vi "TheShooter.vi"() -> ()   [LabVIEW 2019]
uses:
  <vilib>/Rock Robotics/WPI/ThirdParty/Phoenix-LabVIEW/Motor Controller/Controls/CTRE_Phoenix_MotorControl_ControlMode.ctl
  <vilib>/Rock Robotics/WPI/Utilities/WPI_GetSetVariantRefNum.vi
  Robot Global Data.vi
  <vilib>/Rock Robotics/Network Tables/NT Read Number.vi
  <vilib>/Rock Robotics/WPI/ThirdParty/Phoenix-LabVIEW/Motor Controller/Get/CTRE_Phoenix_MotorController_IntegratedSensorData_TalonFX.vi
panel:
  out "shoot state":dbl
  out "Waveform Chart":dbl(graph)
  out "Position":dbl format="%.2f"
  out "MVelocity":dbl
  out "WVelocity":dbl
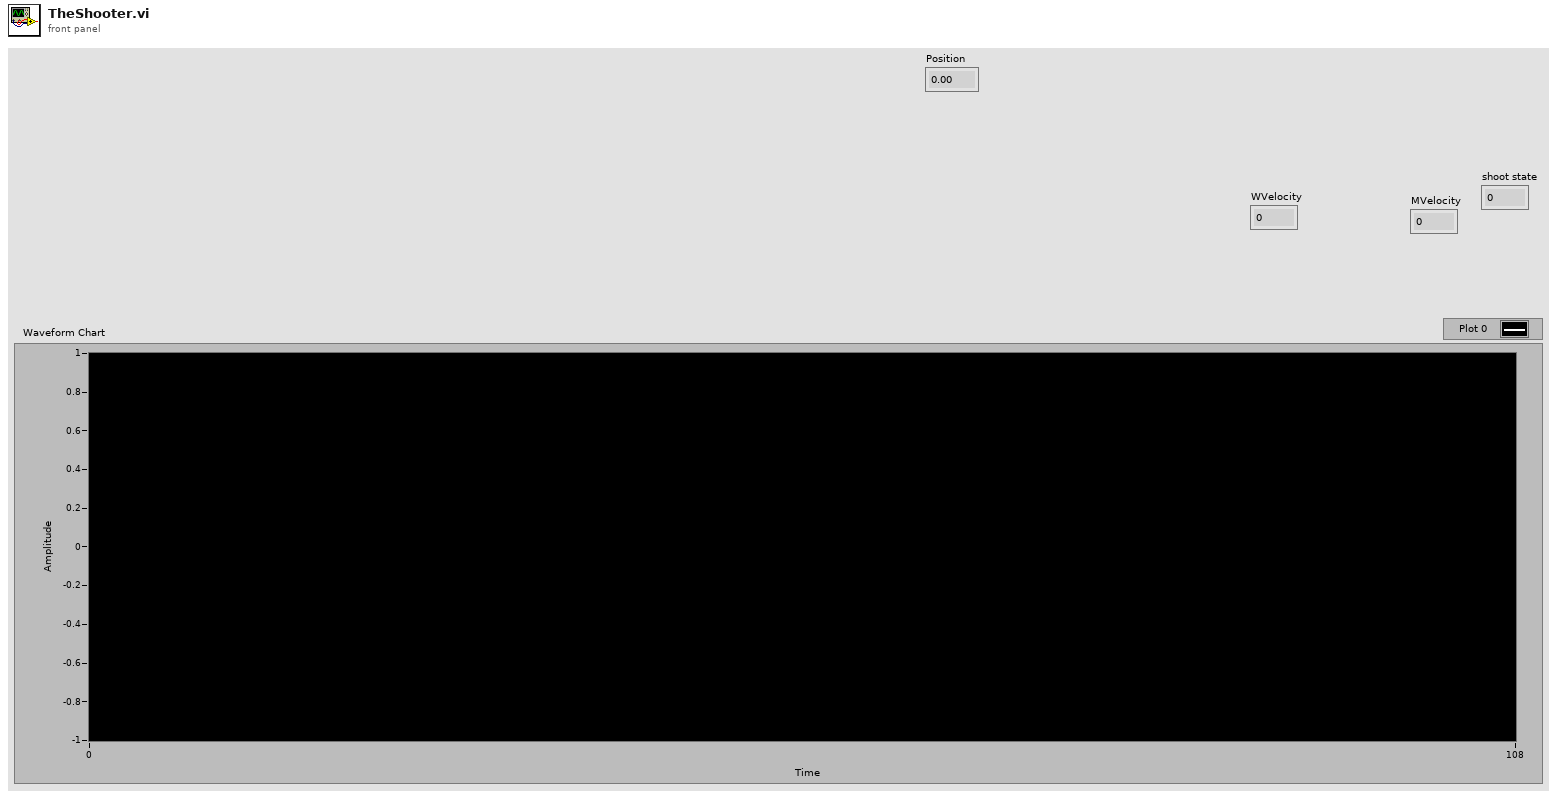
[diagram p1: front panel]
types:
  T1 = typedef "WPI_MotorControlDeviceRef.ctl" = cluster{"DeviceStatus":errorcluster, "Type":T2, "PWM":cluster{"PWM Channel":T3, "DeadBand":T4}, "CAN":cluster{"Device Number":u8, "SetOutput VI Ref":variant, "GetOutput VI Ref":variant, "Enable VI Ref":variant, "Disable VI Ref":variant, "Data":variant}, "Invert":bool, "DIO PWM":cluster{"PWM \"Enable\" Channel":T3, "DIOChannel":T5, "PWM Rate":dbl}}
  T2 = typedef "WPI_MotorControlType.ctl" = enum16{"PWM", "CAN", "DIO PWM"}
  T3 = typedef "FPGA_DIOPWMChannel.ctl" = enum8{"PWM 0", "PWM 1", "PWM 2", "PWM 3", "PWM 4", "PWM 5", "PWM 6", "PWM 7", "PWM 8", "PWM 9", "PWM MXP 0", "PWM MXP 1", "PWM MXP 2", "PWM MXP 3", "PWM MXP 4", "PWM MXP 5", "PWM MXP 6", "PWM MXP 7", "PWM MXP 8", "PWM MXP 9", "Invalid"}
  T4 = typedef "WPI_PWMDeadband.ctl" = cluster{"Name":string, "maxPositivePwm":i32, "minPositivePwm":i32, "centerPwm":i32, "maxNegativePwm":i32, "minNegativePwm":i32, "angularRange":u16}
  T5 = typedef "FPGA_DIOChannel.ctl" = enum8{"DIO 0", "DIO 1", "DIO 2", "DIO 3", "DIO 4", "DIO 5", "DIO 6", "DIO 7", "DIO 8", "DIO 9", "DIO MXP 0", "DIO MXP 1", "DIO MXP 2", "DIO MXP 3", "DIO MXP 4", "DIO MXP 5", "DIO MXP 6", "DIO MXP 7", "DIO MXP 8", "DIO MXP 9", "DIO MXP 10", "DIO MXP 11", "DIO MXP 12", "DIO MXP 13", "DIO MXP 14", "DIO MXP 15", "SPI Port CS1", "SPI Port CS2", "SPI Port CS3", "SPI Port MISO", "SPI Port MOSI", "Invalid"}
  T6 = typedef "WPI_JoystickDevRef.ctl" = cluster{"Device":T7}
  T7 = typedef "WPI_JoystickDeviceEnum.ctl" = enum16{"USB 0", "USB 1", "USB 2", "USB 3", "USB 4", "USB 5"}
  T8 = typedef "CTRE_Phoenix_MotorControl_ControlMode.ctl" = u16
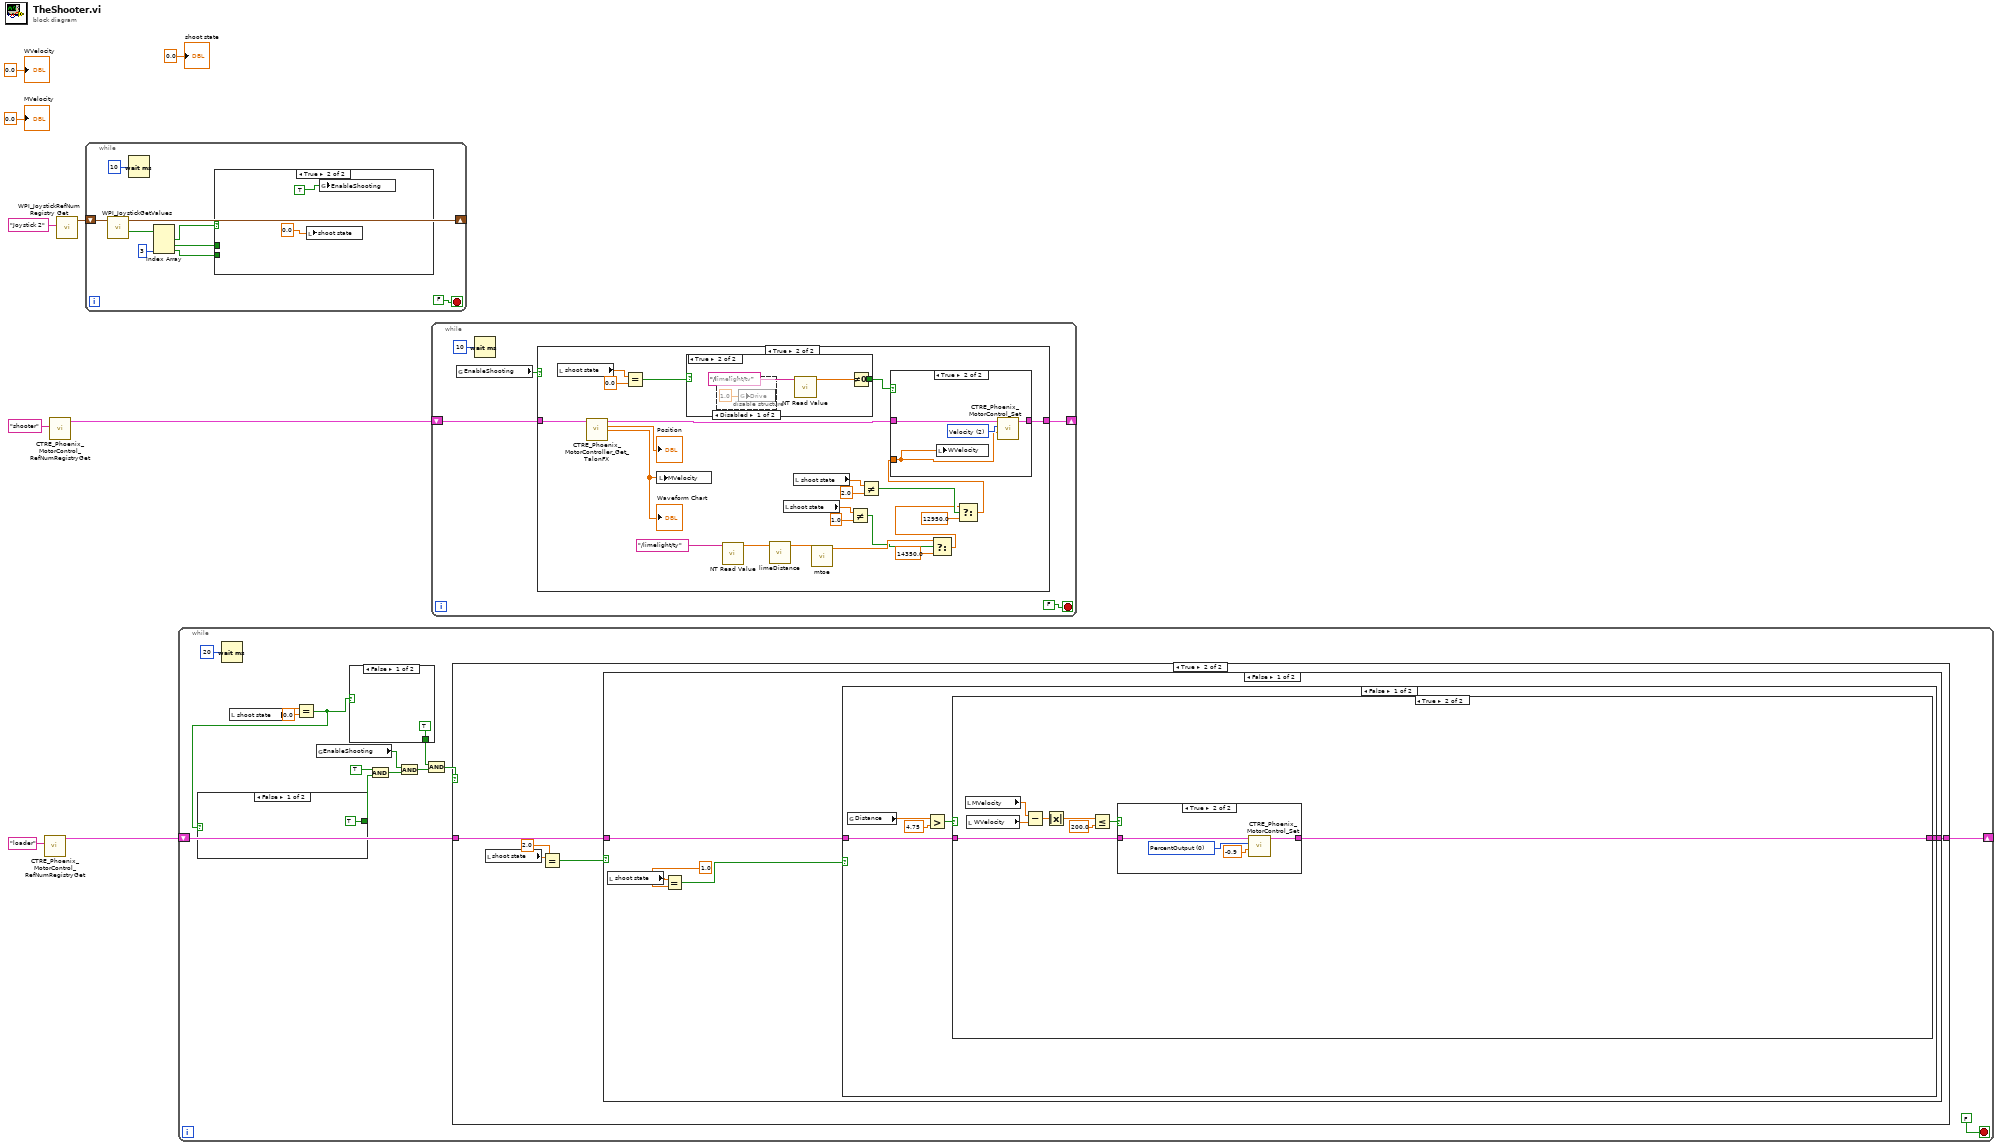
[diagram p0: block diagram]
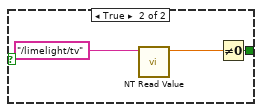
[diagram p2: hidden frame]
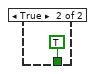
[diagram p3: hidden frame]
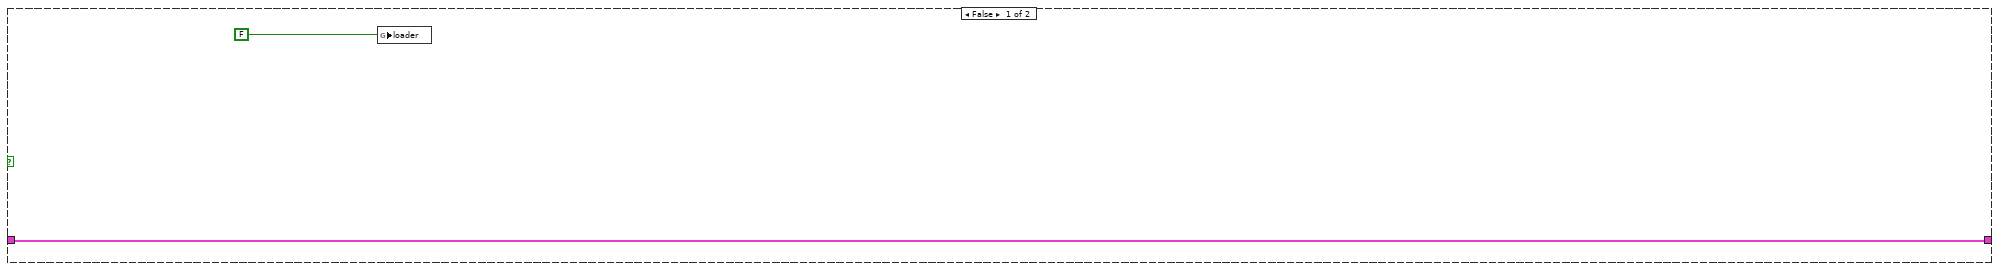
[diagram p4: hidden frame]
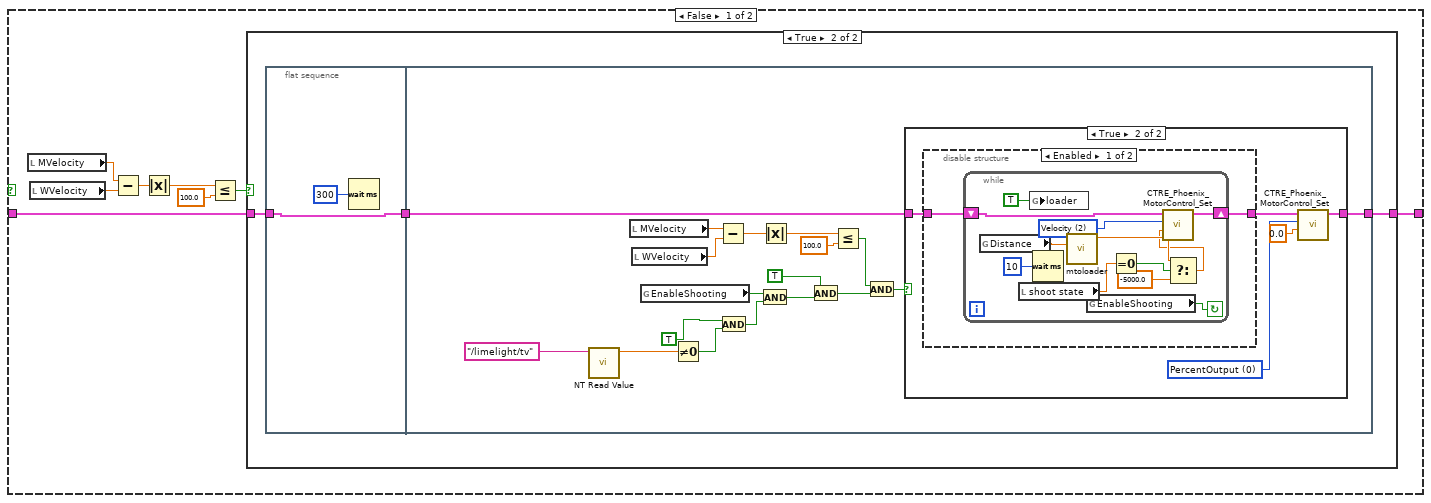
[diagram p5: hidden frame]
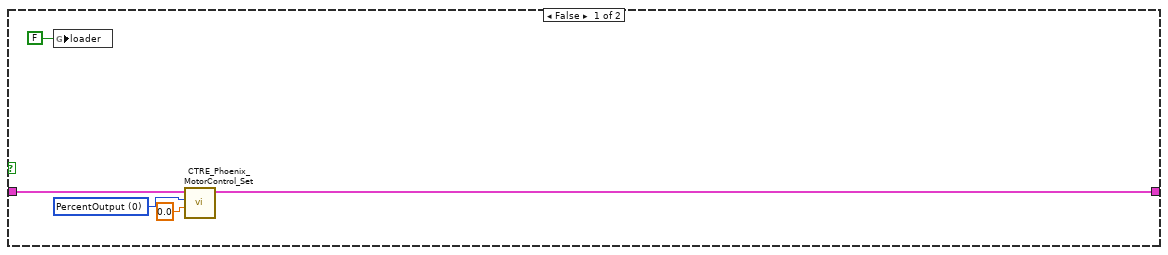
[diagram p6: hidden frame]
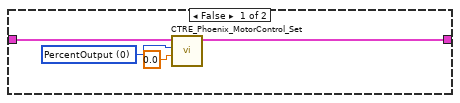
[diagram p7: hidden frame]
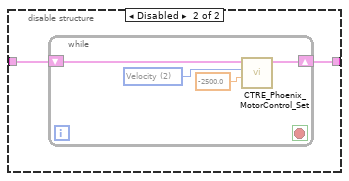
[diagram p8: hidden frame]
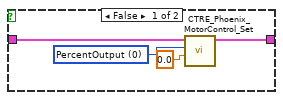
[diagram p9: hidden frame]
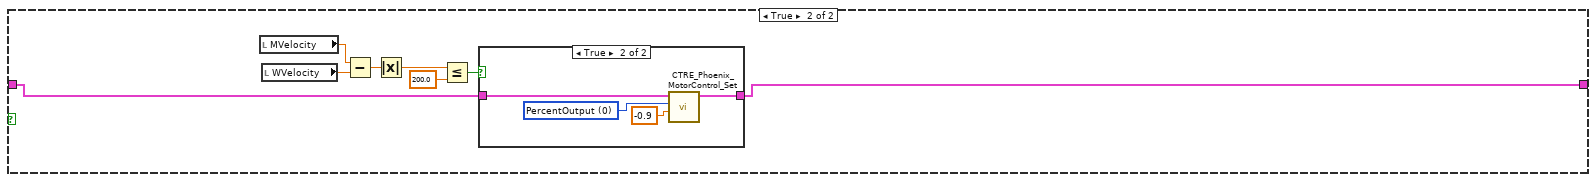
[diagram p10: hidden frame]
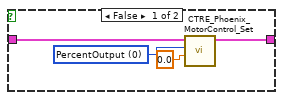
[diagram p11: hidden frame]
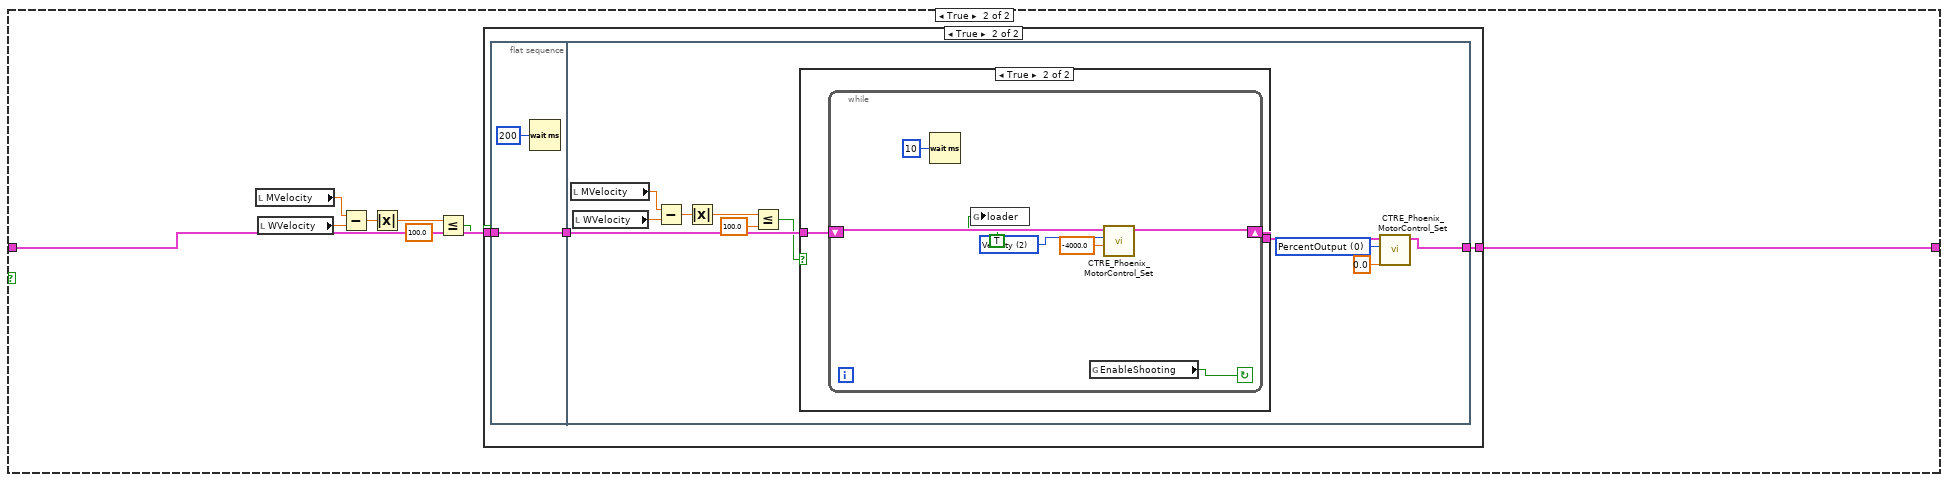
[diagram p12: hidden frame]
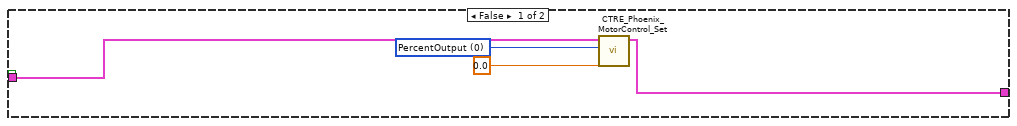
[diagram p13: hidden frame]
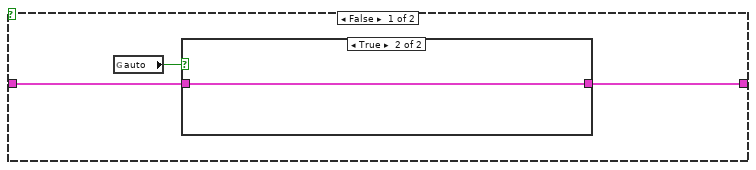
[diagram p15: hidden frame]
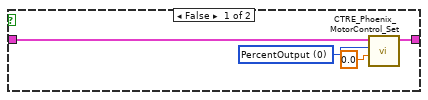
[diagram p16: hidden frame]
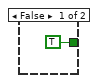
[diagram p17: hidden frame]
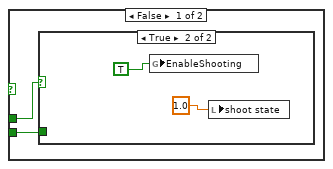
[diagram p20: hidden frame]
diagram:
  n1 = call <vilib>:"CTRE_Phoenix_MotorControl_RefNumRegistryGet.vi"("refnum name"="loader") -> ("PhoenixMotorControlDevRef"=w3:T1)  [unwired: 9 in, 1 out]
  n2 = call <vilib>:"CTRE_Phoenix_MotorControl_RefNumRegistryGet.vi"("refnum name"="shooter") -> ("PhoenixMotorControlDevRef"=w7:T1)  [unwired: 9 in, 1 out]
  n3 = call <vilib>:"WPI_JoystickRefNum Registry Get.vi"("refnum name"="Joystick 2") -> ("JoystickDevRef"=w2:T6)  [unwired: 9 in, 1 out]
  n4 = while {
    shift-right: [w13] -> _
    shift-left: w2 -> [w15]
    stop <- FALSE stop-if-true
    n5 = call <vilib>:"WPI_JoystickGetValues.vi"("JoystickDevRef"=w15) -> ("Buttons"=w18:bool[], "JoystickDevRef"=w13:T6)  [unwired: 6 in, 3 out]
    n6 = Wait (ms)(milliseconds to wait=u32 10) -> ()  [unwired: 1 out]
    n7 = Index Array(array=w18, index #3=3 ("index")) -> (element #1=w12:bool, element #2=w11:bool, element #3=w10:bool)  [unwired: 2 in]
    n8 = case shown="True" w12 {
      tunnel: w11 -> [w20 _]
      tunnel: w10 -> [w19 _]
      frame False {
        n9 = case shown="True" w20 {
          tunnel: w19 -> [w21 _]
          frame False {
            n10 = case shown="True" w21 {
              frame False {
                n11 = global read "Robot Global Data.vi" "auto"() -> (w22:bool)
                n12 = case shown="False" w22 {
                  frame False {
                    n13 = global write "Robot Global Data.vi" "EnableShooting"(FALSE ("EnableShooting")) -> ()
                  }
                  frame True {
                  }
                }
              }
              frame True {
                n14 = global write "Robot Global Data.vi" "EnableShooting"(TRUE ("EnableShooting")) -> ()
                n15 = local write "shoot state"(2.0 ("Loader")) -> ()
              }
            }
          }
          frame True {
            n16 = global write "Robot Global Data.vi" "EnableShooting"(TRUE ("EnableShooting")) -> ()
            n17 = local write "shoot state"(1.0 ("Loader")) -> ()
          }
        }
      }
      frame True {
        n18 = local write "shoot state"(0.0 ("Loader")) -> ()
        n19 = global write "Robot Global Data.vi" "EnableShooting"(TRUE ("EnableShooting")) -> ()
      }
    }
  }
  n20 = while {
    shift-right: [w41] -> _
    shift-left: w3 -> [w42]
    stop <- FALSE stop-if-true
    n21 = Wait (ms)(milliseconds to wait=u32 20) -> ()  [unwired: 1 out]
    n22 = local read "shoot state"() -> (w33:dbl)
    n23 = Equal?(x=w33, y=0.0) -> (x = y?=w31:bool)
    n24 = case shown="False" w31 {
      tunnel: [TRUE w45] -> w35
      frame False {
      }
      frame True {
        n25 = call-poly <vilib>:"NT Read Value.vi"("Name"="/limelight/tv") -> ("Numeric"=w46:dbl)  [unwired: 9 in, 1 out]
        n26 = Not Equal To 0?(x=w46) -> (x != 0?=w45:bool)
      }
    }
    n27 = global read "Robot Global Data.vi" "EnableShooting"() -> (w37:bool)
    n28 = case shown="False" w31 {
      tunnel: [TRUE ("In Angle") TRUE ("In Angle")] -> w38
      frame False {
      }
      frame True {
      }
    }
    n29 = And(x=TRUE, y=w35) -> (x .and. y?=w34:bool)
    n30 = And(x=w37, y=w34) -> (x .and. y?=w36:bool)
    n31 = And(x=w38, y=w36) -> (x .and. y?=w39:bool)
    n32 = case shown="True" w39 {
      tunnel: w42 -> [w51 w55]
      tunnel: [w51 w56] -> w41
      frame False {
        n33 = global write "Robot Global Data.vi" "loader"(FALSE ("If loaderMoves")) -> ()
      }
      frame True {
        n34 = local read "shoot state"() -> (w54:dbl)
        n35 = Equal?(x=w54, y=2.0) -> (x = y?=w52:bool)
        n36 = case shown="False" w52 {
          tunnel: [w61 w170] -> w56
          tunnel: w55 -> [w60 w171]
          frame False {
            n37 = local read "shoot state"() -> (w59:dbl)
            n38 = Equal?(x=w59, y=1.0) -> (x = y?=w57:bool)
            n39 = case shown="False" w57 {
              tunnel: [w66 w148] -> w61
              tunnel: w60 -> [w65 w149]
              frame False {
                n40 = global read "Robot Global Data.vi" "Distance"() -> (w64:dbl)
                n41 = Greater?(x=w64, y=4.75) -> (0:w62:bool)
                n42 = case shown="True" w62 {
                  tunnel: [w69 w132] -> w66
                  tunnel: w65 -> [w67 w133]
                  frame False {
                    n43 = local read "MVelocity"() -> (w73:dbl)
                    n44 = local read "WVelocity"() -> (w72:dbl)
                    n45 = Subtract(x=w73, y=w72) -> (x-y=w71:dbl)
                    n46 = Absolute Value(x=w71) -> (abs(x)=w70:dbl)
                    n47 = Less Or Equal?(x=w70, y=100.0) -> (x <= y?=w68:bool)
                    n48 = case shown="True" w68 {
                      tunnel: w67 -> [w77 w82]
                      tunnel: [w76 w81] -> w69
                      frame False {
                        w79 = T8 0 items=["PercentOutput"=0, "Position"=1, "Velocity"=2, "Current"=3, "Follower"=5, "MotionProfile"=6, "MotionMagic"=7, "MotionProfileArc"=10, "Disabled"=15] ("Control Mode")
                        n49 = global write "Robot Global Data.vi" "loader"(FALSE ("If loaderMoves")) -> ()
                        n50 = call <vilib>:"CTRE_Phoenix_MotorControl_Set.vi"("Output"=0.0, "Control Mode"=w79, "PhoenixMotorControlDevRef"=w77) -> ("PhoenixMotorControlDevRef"=w76:T1)  [unwired: 7 in, 1 out]
                      }
                      frame True {
                        n51 = flat-sequence {
                          tunnel: w82 -> [w84]
                          tunnel: [w84] -> w80
                          tunnel: [w101] -> w81
                          tunnel: w80 -> [w102]
                          frame #0 {
                            n52 = Wait (ms)(milliseconds to wait=u32 300) -> ()  [unwired: 1 out]
                          }
                          frame #1 {
                            n53 = call-poly <vilib>:"NT Read Value.vi"("Name"="/limelight/tv") -> ("Numeric"=w90:dbl)  [unwired: 9 in, 1 out]
                            n54 = local read "MVelocity"() -> (w97:dbl)
                            n55 = local read "WVelocity"() -> (w98:dbl)
                            n56 = global read "Robot Global Data.vi" "EnableShooting"() -> (w92:bool)
                            n57 = Not Equal To 0?(x=w90) -> (x != 0?=w91:bool)
                            n58 = Subtract(x=w97, y=w98) -> (x-y=w99:dbl)
                            n59 = And(x=TRUE, y=w91) -> (x .and. y?=w88:bool)
                            n60 = And(x=w92, y=w88) -> (x .and. y?=w93:bool)
                            n61 = Absolute Value(x=w99) -> (abs(x)=w100:dbl)
                            n62 = And(x=TRUE, y=w93) -> (x .and. y?=w87:bool)
                            n63 = Less Or Equal?(x=w100, y=100.0) -> (x <= y?=w95:bool)
                            n64 = And(x=w95, y=w87) -> (x .and. y?=w94:bool)
                            n65 = case shown="True" w94 {
                              tunnel: w102 -> [w106 w111]
                              tunnel: [w105 w110] -> w101
                              frame False {
                                w104 = T8 0 items=["PercentOutput"=0, "Position"=1, "Velocity"=2, "Current"=3, "Follower"=5, "MotionProfile"=6, "MotionMagic"=7, "MotionProfileArc"=10, "Disabled"=15] ("Control Mode")
                                n66 = call <vilib>:"CTRE_Phoenix_MotorControl_Set.vi"("Output"=0.0, "Control Mode"=w104, "PhoenixMotorControlDevRef"=w106) -> ("PhoenixMotorControlDevRef"=w105:T1)  [unwired: 7 in, 1 out]
                              }
                              frame True {
                                w108 = T8 0 items=["PercentOutput"=0, "Position"=1, "Velocity"=2, "Current"=3, "Follower"=5, "MotionProfile"=6, "MotionMagic"=7, "MotionProfileArc"=10, "Disabled"=15] ("Control Mode")
                                n67 = disable-structure shown="Enabled" {
                                disable-tunnel: w111 -> [w113 w126]
                                disable-tunnel: [w112 w127] -> w109
                                frame Enabled {
                                n68 = while {
                                shift-right: [w123] -> w112
                                shift-left: w113 -> [w124]
                                stop <- w121 continue-if-true
                                w125 = T8 2 items=["PercentOutput"=0, "Position"=1, "Velocity"=2, "Current"=3, "Follower"=5, "MotionProfile"=6, "MotionMagic"=7, "MotionProfileArc"=10, "Disabled"=15] ("Control Mode")
                                n69 = global read "Robot Global Data.vi" "Distance"() -> (w119:dbl)
                                n70 = local read "shoot state"() -> (w114:dbl)
                                n71 = global write "Robot Global Data.vi" "loader"(TRUE ("If loaderMoves")) -> ()
                                n72 = Wait (ms)(milliseconds to wait=u32 10) -> ()  [unwired: 1 out]
                                n73 = call "mtoloader.vi"("m"=w119) -> ("loader"=w118:dbl)  [unwired: 10 in]
                                n74 = global read "Robot Global Data.vi" "EnableShooting"() -> (w121:bool)
                                n75 = Equal To 0?(x=w114) -> (x = 0?=w115:bool)
                                n76 = Select(t=w118, s=w115, f=-5000.0) -> (s? t:f=w117:dbl)
                                n77 = call <vilib>:"CTRE_Phoenix_MotorControl_Set.vi"("Output"=w117, "Control Mode"=w125, "PhoenixMotorControlDevRef"=w124) -> ("PhoenixMotorControlDevRef"=w123:T1)  [unwired: 7 in, 1 out]
                                }
                                }
                                frame Disabled {
                                n78 = while {
                                shift-right: [w131] -> w127
                                shift-left: w126 -> [w130]
                                stop <- _ stop-if-true
                                w129 = T8 2 items=["PercentOutput"=0, "Position"=1, "Velocity"=2, "Current"=3, "Follower"=5, "MotionProfile"=6, "MotionMagic"=7, "MotionProfileArc"=10, "Disabled"=15] ("Control Mode")
                                n79 = call <vilib>:"CTRE_Phoenix_MotorControl_Set.vi"("Output"=-2500.0, "Control Mode"=w129, "PhoenixMotorControlDevRef"=w130) -> ("PhoenixMotorControlDevRef"=w131:T1)  [unwired: 7 in, 1 out]
                                }
                                }
                                }
                                n80 = call <vilib>:"CTRE_Phoenix_MotorControl_Set.vi"("Output"=0.0, "Control Mode"=w108, "PhoenixMotorControlDevRef"=w109) -> ("PhoenixMotorControlDevRef"=w110:T1)  [unwired: 7 in, 1 out]
                              }
                            }
                          }
                        }
                      }
                    }
                  }
                  frame True {
                    n81 = local read "MVelocity"() -> (w139:dbl)
                    n82 = local read "WVelocity"() -> (w138:dbl)
                    n83 = Subtract(x=w139, y=w138) -> (x-y=w137:dbl)
                    n84 = Absolute Value(x=w137) -> (abs(x)=w136:dbl)
                    n85 = Less Or Equal?(x=w136, y=200.0) -> (x <= y?=w134:bool)
                    n86 = case shown="True" w134 {
                      tunnel: w133 -> [w143 w147]
                      tunnel: [w142 w146] -> w132
                      frame False {
                        w141 = T8 0 items=["PercentOutput"=0, "Position"=1, "Velocity"=2, "Current"=3, "Follower"=5, "MotionProfile"=6, "MotionMagic"=7, "MotionProfileArc"=10, "Disabled"=15] ("Control Mode")
                        n87 = call <vilib>:"CTRE_Phoenix_MotorControl_Set.vi"("Output"=0.0, "Control Mode"=w141, "PhoenixMotorControlDevRef"=w143) -> ("PhoenixMotorControlDevRef"=w142:T1)  [unwired: 7 in, 1 out]
                      }
                      frame True {
                        w145 = T8 0 items=["PercentOutput"=0, "Position"=1, "Velocity"=2, "Current"=3, "Follower"=5, "MotionProfile"=6, "MotionMagic"=7, "MotionProfileArc"=10, "Disabled"=15] ("Control Mode")
                        n88 = call <vilib>:"CTRE_Phoenix_MotorControl_Set.vi"("Output"=-0.9, "Control Mode"=w145, "PhoenixMotorControlDevRef"=w147) -> ("PhoenixMotorControlDevRef"=w146:T1)  [unwired: 7 in, 1 out]
                      }
                    }
                  }
                }
              }
              frame True {
                n89 = local read "MVelocity"() -> (w155:dbl)
                n90 = local read "WVelocity"() -> (w154:dbl)
                n91 = Subtract(x=w155, y=w154) -> (x-y=w153:dbl)
                n92 = Absolute Value(x=w153) -> (abs(x)=w152:dbl)
                n93 = Less Or Equal?(x=w152, y=200.0) -> (x <= y?=w151:bool)
                n94 = case shown="True" w151 {
                  tunnel: w149 -> [w159 w163]
                  tunnel: [w158 w162] -> w148
                  frame False {
                    w157 = T8 0 items=["PercentOutput"=0, "Position"=1, "Velocity"=2, "Current"=3, "Follower"=5, "MotionProfile"=6, "MotionMagic"=7, "MotionProfileArc"=10, "Disabled"=15] ("Control Mode")
                    n95 = call <vilib>:"CTRE_Phoenix_MotorControl_Set.vi"("Output"=0.0, "Control Mode"=w157, "PhoenixMotorControlDevRef"=w159) -> ("PhoenixMotorControlDevRef"=w158:T1)  [unwired: 7 in, 1 out]
                  }
                  frame True {
                    w161 = T8 0 items=["PercentOutput"=0, "Position"=1, "Velocity"=2, "Current"=3, "Follower"=5, "MotionProfile"=6, "MotionMagic"=7, "MotionProfileArc"=10, "Disabled"=15] ("Control Mode")
                    n96 = call <vilib>:"CTRE_Phoenix_MotorControl_Set.vi"("Output"=-0.9, "Control Mode"=w161, "PhoenixMotorControlDevRef"=w163) -> ("PhoenixMotorControlDevRef"=w162:T1)  [unwired: 7 in, 1 out]
                  }
                }
              }
            }
          }
          frame True {
            n97 = local read "MVelocity"() -> (w169:dbl)
            n98 = local read "WVelocity"() -> (w168:dbl)
            n99 = Subtract(x=w169, y=w168) -> (x-y=w167:dbl)
            n100 = Absolute Value(x=w167) -> (abs(x)=w166:dbl)
            n101 = Less Or Equal?(x=w166, y=100.0) -> (x <= y?=w164:bool)
            n102 = case shown="True" w164 {
              tunnel: w171 -> [w173 w178]
              tunnel: [w172 w177] -> w170
              frame False {
                w175 = T8 0 items=["PercentOutput"=0, "Position"=1, "Velocity"=2, "Current"=3, "Follower"=5, "MotionProfile"=6, "MotionMagic"=7, "MotionProfileArc"=10, "Disabled"=15] ("Control Mode")
                n103 = call <vilib>:"CTRE_Phoenix_MotorControl_Set.vi"("Output"=0.0, "Control Mode"=w175, "PhoenixMotorControlDevRef"=w173) -> ("PhoenixMotorControlDevRef"=w172:T1)  [unwired: 7 in, 1 out]
              }
              frame True {
                n104 = flat-sequence {
                  tunnel: w178 -> [w180]
                  tunnel: [w180] -> w176
                  tunnel: [w189] -> w177
                  tunnel: w176 -> [w191]
                  frame #0 {
                    n105 = Wait (ms)(milliseconds to wait=u32 200) -> ()  [unwired: 1 out]
                  }
                  frame #1 {
                    w188 = T8 0 items=["PercentOutput"=0, "Position"=1, "Velocity"=2, "Current"=3, "Follower"=5, "MotionProfile"=6, "MotionMagic"=7, "MotionProfileArc"=10, "Disabled"=15] ("Control Mode")
                    n106 = local read "MVelocity"() -> (w182:dbl)
                    n107 = local read "WVelocity"() -> (w183:dbl)
                    n108 = Subtract(x=w182, y=w183) -> (x-y=w184:dbl)
                    n109 = Absolute Value(x=w184) -> (abs(x)=w185:dbl)
                    n110 = Less Or Equal?(x=w185, y=100.0) -> (x <= y?=w181:bool)
                    n111 = case shown="True" w181 {
                      tunnel: w191 -> [w192 w194]
                      tunnel: [w192 w193] -> w190
                      frame False {
                      }
                      frame True {
                        n112 = while {
                          shift-right: [w197] -> w193
                          shift-left: w194 -> [w198]
                          stop <- w201 continue-if-true
                          w200 = T8 2 items=["PercentOutput"=0, "Position"=1, "Velocity"=2, "Current"=3, "Follower"=5, "MotionProfile"=6, "MotionMagic"=7, "MotionProfileArc"=10, "Disabled"=15] ("Control Mode")
                          n113 = Wait (ms)(milliseconds to wait=u32 10) -> ()  [unwired: 1 out]
                          n114 = global write "Robot Global Data.vi" "loader"(TRUE ("loader")) -> ()
                          n115 = global read "Robot Global Data.vi" "EnableShooting"() -> (w201:bool)
                          n116 = call <vilib>:"CTRE_Phoenix_MotorControl_Set.vi"("Output"=-4000.0, "Control Mode"=w200, "PhoenixMotorControlDevRef"=w198) -> ("PhoenixMotorControlDevRef"=w197:T1)  [unwired: 7 in, 1 out]
                        }
                      }
                    }
                    n117 = call <vilib>:"CTRE_Phoenix_MotorControl_Set.vi"("Output"=0.0, "Control Mode"=w188, "PhoenixMotorControlDevRef"=w190) -> ("PhoenixMotorControlDevRef"=w189:T1)  [unwired: 7 in, 1 out]
                  }
                }
              }
            }
          }
        }
      }
    }
  }
  n118 = while {
    shift-right: [w204] -> _
    shift-left: w7 -> [w205]
    stop <- FALSE stop-if-true
    n119 = global read "Robot Global Data.vi" "EnableShooting"() -> (w202:bool)
    n120 = Wait (ms)(milliseconds to wait=u32 10) -> ()  [unwired: 1 out]
    n121 = case shown="True" w202 {
      tunnel: w205 -> [w209 w236]
      tunnel: [w208 w237] -> w204
      frame False {
        n122 = global read "Robot Global Data.vi" "auto"() -> (w207:bool)
        n123 = case shown="True" w207 {
          tunnel: w209 -> [w213 w214]
          tunnel: [w212 w214] -> w208
          frame False {
            w211 = T8 0 items=["PercentOutput"=0, "Position"=1, "Velocity"=2, "Current"=3, "Follower"=5, "MotionProfile"=6, "MotionMagic"=7, "MotionProfileArc"=10, "Disabled"=15] ("Control Mode")
            n124 = call <vilib>:"CTRE_Phoenix_MotorControl_Set.vi"("Output"=0.0, "Control Mode"=w211, "PhoenixMotorControlDevRef"=w213) -> ("PhoenixMotorControlDevRef"=w212:T1)  [unwired: 7 in, 1 out]
          }
          frame True {
          }
        }
      }
      frame True {
        n125 = local read "shoot state"() -> (w222:dbl)
        n126 = call-poly <vilib>:"CTRE_Phoenix_MotorController_Get_TalonFX.vi"("PhoenixMotorControlDevRef"=w236) -> ("PhoenixMotorControlDevRef"=w233:T1, "Position"=→"Position":dbl, "Velocity"=w232:dbl)  [unwired: 10 in, 2 out]
        "Waveform Chart" <- w232
        n127 = Equal?(x=w222, y=0.0) -> (x = y?=w221:bool)
        n128 = local write "MVelocity"(w232) -> ()
        n129 = case shown="True" w221 {
          tunnel: [TRUE w240] -> w229
          frame False {
          }
          frame True {
            n130 = disable-structure shown="Disabled" {
              frame Disabled {
                n131 = global write "Robot Global Data.vi" "Drive"(1.0 ("Drive")) -> ()
              }
              frame Enabled {
              }
            }
            n132 = call-poly <vilib>:"NT Read Value.vi"("Name"="/limelight/tv") -> ("Numeric"=w239:dbl)  [unwired: 9 in, 1 out]
            n133 = Not Equal To 0?(x=w239) -> (x != 0?=w240:bool)
          }
        }
        n134 = call-poly <vilib>:"NT Read Value.vi"("Name"="/limelight/ty") -> ("Numeric"=w231:dbl)  [unwired: 9 in, 1 out]
        n135 = call "limeDistance.vi"("a2"=w231) -> ("d"=w230:dbl)  [unwired: 10 in]
        n136 = local read "shoot state"() -> (w219:dbl)
        n137 = local read "shoot state"() -> (w228:dbl)
        n138 = call "mtoe.vi"("m"=w230) -> ("e"=w218:dbl)  [unwired: 10 in]
        n139 = Not Equal?(x=w219, y=1.0) -> (x != y?=w216:bool)
        n140 = Not Equal?(x=w228, y=2.0) -> (x != y?=w226:bool)
        n141 = Select(t=w218, s=w216, f=14350.0) -> (s? t:f=w217:dbl)
        n142 = Select(t=w217, s=w226, f=12950.0) -> (s? t:f=w225:dbl)
        n143 = case shown="True" w229 {
          tunnel: w233 -> [w243 w246]
          tunnel: [w243 w245] -> w237
          tunnel: w225 -> [_ w244]
          frame False {
          }
          frame True {
            w247 = T8 2 items=["PercentOutput"=0, "Position"=1, "Velocity"=2, "Current"=3, "Follower"=5, "MotionProfile"=6, "MotionMagic"=7, "MotionProfileArc"=10, "Disabled"=15] ("Control Mode")
            n144 = local write "WVelocity"(w244) -> ()
            n145 = call <vilib>:"CTRE_Phoenix_MotorControl_Set.vi"("Output"=w244, "Control Mode"=w247, "PhoenixMotorControlDevRef"=w246) -> ("PhoenixMotorControlDevRef"=w245:T1)  [unwired: 7 in, 1 out]
          }
        }
      }
    }
  }
  "WVelocity" <- 0.0 ("MVelocity")
  "MVelocity" <- 0.0 ("MVelocity")
  "shoot state" <- 0.0 ("MVelocity")
